vi "AsyncEngine.CANProtectionAndCounter.vi"(10 "Parameters":variant, 11 "Process":refnum<class "Process.lvclass">) -> ()   [LabVIEW 2019, in "Protection and Counter Addon Engine.lvlib"]
uses:
  Protection and Counter Addon Engine.lvlib
  <vilib>/NI/NIVS Inline Async API/_VS Inline Async API/Process/Process.lvclass
  Types/RT Async Engine Settings.ctl
  SubModules/Frame Protection Support/Source/Engine/Types/RT Frame Settings.ctl
  SubModules/Frame Protection Support/Source/Shared/Types/Exported Frame Type.ctl
  SubModules/Frame Protection Support/Source/Engine/Types/RT Protection Configuration.ctl
  SubModules/Frame Protection Support/Source/Shared/Types/Protection Type.ctl
  SubModules/Frame Protection Support/Source/Shared/Types/XNET Signal Configuration.ctl
  SubModules/Frame Protection Support/Source/Shared/Types/Exported Counter Settings.ctl
  SubModules/Frame Protection Support/Source/Shared/Types/Exported Event Trigger Type.ctl
  <vilib>/Platform/TimedLoop/XDataNode/timing_clust.ctl
  <vilib>/Platform/TimedLoop/XDataNode/nitl_modes.ctl
  <vilib>/Platform/TimedLoop/XDataNode/wakeup.ctl
  <vilib>/NI/NIVS Inline Async API/_Data Access Engine/Access Type Classes/Read/Read.lvclass/Read.ctl
  <vilib>/NI/NIVS Inline Async API/_Data Access Engine/Access Type Classes/Write/Write.lvclass/Write.ctl
  <vilib>/NI/NIVS Inline Async API/_VS Inline Async API/Process/Process.lvclass/Process.ctl
  <vilib>/NI/NIVS Inline Async API/_VS Inline Async API/Error Handling Process/SubVIs/Error.ConvertArray.vi
  <vilib>/NI/NIVS Inline Async API/_Data Access Engine/Data Access Engine/Methods/Data.Processes.Execute.vi
  <vilib>/NI/NIVS Inline Async API/_Data Access Engine/Data Access Engine/Methods/Write.Data.vi
  SubModules/Frame Protection Support/Source/Engine/SubVIs/Calculate Counter And Protections Main.vi
  <vilib>/NI/NIVS Inline Async API/_Data Access Engine/Access Type Classes/Write/Write.ProcessData.vi
  <vilib>/NI/NIVS Inline Async API/_Data Access Engine/Data Access Engine/Methods/Read.Data.Detect.vi
  SubModules/Frame Protection Support/Source/Engine/SubVIs/Determine Transmit.vi
  SubModules/Frame Protection Support/Source/Engine/SubVIs/Update Counter Signals.vi
  SubModules/Frame Protection Support/Source/Engine/SubVIs/Get Frame Data.vi
  SubModules/Frame Protection Support/Source/Engine/SubVIs/Convert EU Data to XNET Frame.vi
  SubModules/Frame Protection Support/Source/Engine/SubVIs/Update Protection Signals.vi
  SubModules/Frame Protection Support/Source/Engine/SubVIs/Determine Disabled.vi
  <vilib>/NI/NIVS Inline Async API/_Data Access Engine/Data Access Engine/Methods/Write.Data.Commit.vi
  <vilib>/NI/NIVS Inline Async API/_Data Access Engine/Access Type Classes/Write/Write.Buffer.vi
  <vilib>/NI/NIVS Inline Async API/_Data Access Engine/Access Type Classes/Write/Write.Commit.vi
  <vilib>/NI/NIVS Inline Async API/_Data Access Engine/Access Type Classes/Read/Read.ProcessData.Detect.vi
  SubModules/Frame Protection Support/Source/Engine/SubVIs/Determine Transmission.vi
  SubModules/Frame Protection Support/Source/Engine/SubVIs/Determine Periodic.vi
  SubModules/Frame Protection Support/Source/Engine/SubVIs/Set Counter Signal.vi
  SubModules/Frame Protection Support/Source/Engine/SubVIs/Calculate Counter Value.vi
  SubModules/Frame Protection Support/Source/Engine/SubVIs/Set Protection Signal.vi
  SubModules/Frame Protection Support/Source/Engine/SubVIs/Calculate Protection Value.vi
  <vilib>/NI/NIVS Inline Async API/_Data Access Engine/Data Access Engine/Methods/Write.Data.Buffer.vi
  SubModules/Frame Protection Support/Source/Engine/SubVIs/Get Protection Signals.vi
  <vilib>/xnet/xnet.llb/XNET Convert.vi
  <vilib>/xnet/xnet.llb/XNET Convert (Signal to Frame Raw).vi
  <vilib>/xnet/xnet.llb/XNET Convert (Signal to Frame CAN).vi
  <vilib>/xnet/xnet.llb/XNET Write.vi
  <vilib>/xnet/xnet.llb/XNET Write (Frame CAN).vi
  <vilib>/NI/NI VeriStand Addon Network Comm/Engine/VeriStand Comm.lvclass
  <vilib>/NI/NIVS Inline Async API/_Data Access Engine/Access Type Classes/Write/Write.lvclass
  <vilib>/NI/NIVS Inline Async API/_Data Access Engine/Access Type Classes/Read/Read.lvclass
  <vilib>/Platform/TimedLoop/XDataNode/XDataNode.xnode
  SubModules/Frame Protection Support/Source/Shared/Protection and Counter Support Shared.lvlib
  SubModules/Frame Protection Support/Source/Engine/Protection and Counter Support Engine.lvlib
  <vilib>/Platform/TimedLoop/XDataNode/XDNodeRunTimeDep.lvlib
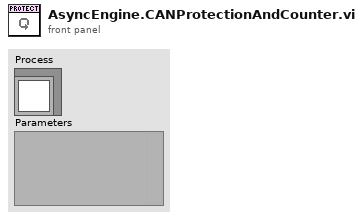
[diagram p1: front panel]
types:
  T1 = typedef "Protection and Counter Addon Engine.lvlib/RT Async Engine Settings.ctl" = cluster{"Name":string, "Priority":i32, "CAN Session":refnum<k21>, "Frame Count":i32, "Frames":T2[], "FPGA Session":u32}
  T2 = typedef "Protection and Counter Support Engine.lvlib/RT Frame Settings.ctl" = cluster{"Type":T3, "Frame ID":u32, "Payload Length":u32, "VS Offset":i32, "VS Length":i32, "Frame Conversion":refnum<k21>, "Frame.Data":dbl[], "Generation Period":u32, "Time Since Last Generation":u32, "Generation Iterations":u32, "Generation Counter":u32, "Has Protection?":bool, "Protection Configurations":T4[], "Has Counter?":bool, "Counter Configurations":T7[], "Has Disable?":bool, "Disable VS Index":i32, "Transmit Trigger":T8, "Trigger VS Index":i32}
  T3 = typedef "Protection and Counter Support Shared.lvlib/Exported Frame Type.ctl" = enum16{"Periodic", "Event", "Periodic/Event"}
  T4 = typedef "Protection and Counter Support Engine.lvlib/RT Protection Configuration.ctl" = cluster{"Protection Frame Index":i32, "Protection Type":T5, "Data Indeces":i32[], "Data Array":dbl[], "Check Sum Conversion":refnum<k21>, "CRC Channels":T6[], "Protection VS Index":i32, "Counter Data Index":i32}
  T5 = typedef "Protection and Counter Support Shared.lvlib/Protection Type.ctl" = enum16{"Arb ID + Bytes Checksum with Inversion", "Arb ID + Bytes CRC with Inversion", "Reversed Raw Signal Checksum with Inversion", "Concatenated Two's Compliment"}
  T6 = typedef "Protection and Counter Support Shared.lvlib/XNET Signal Configuration.ctl" = cluster{"Start Bit":i32, "Name":string, "Number of bits":i32, "Scale":dbl, "Offset":dbl, "Data Type":u32, "Counter":bool}
  T7 = typedef "Protection and Counter Support Shared.lvlib/Exported Counter Settings.ctl" = cluster{"Frame Index":i32, "Max Count":dbl, "VS Index":i32, "Bit Length":i64}
  T8 = typedef "Protection and Counter Support Shared.lvlib/Exported Event Trigger Type.ctl" = enum16{"Channel value change", "Trigger channel (not zero)", "Channel value change or trigger channel (not zero)", "Trigger channel (any value change)", "Channel value change or trigger channel (any value change)"}
  T9 = typedef "Protection and Counter Addon Engine.lvlib/RT Async Engine Variables.ctl" = cluster{"Process Ref":refnum<class "Process.lvclass">, "Comm Ref":refnum<class "VeriStand Comm.lvclass">, "Data Refs":T10, "Settings":T1}
  T10 = typedef "Protection and Counter Addon Engine.lvlib/RT Data References.ctl" = cluster{"ProtectionsAndCounters.Ref":T11, "Signals.Ref":T12, "Status.Ref":T11}
  T11 = typedef "Data Access Engine.lvlib/Data Access Engine.lvclass/Write.DVR.ctl" = refnum<data-value>
  T12 = typedef "Data Access Engine.lvlib/Data Access Engine.lvclass/Read.DVR.ctl" = refnum<data-value>
  T13 = typedef "XDNodeRunTimeDep.lvlib/timing_clust.ctl" = cluster{"Expected End [f-1]":u64, "Actual End [f-1]":u64, "Finished Late? [f-1]":bool, "Expected End [i-1]":u64, "Actual End [i-1]":u64, "Finished Late? [i-1]":bool, "Expected Start [i]":u64, "Actual Start [i]":u64, "Expected Start [f]":u64, "Actual Start [f]":u64, "Source Name":string, "Structure Name":string, "Period":i64, "Deadline":i64, "Offset":i64, "Start":i64, "Priority":i32, "Timeout":i32, "Mode":T14, "Wakeup Reason":T15, "Error":errorcluster, "Source Type":string, "Secondary Source Type":string, "Global End Time":u64, "Global Start Time":u64, "Frame Duration":u64, "Iteration Duration":u64, "Assigned CPU":i32, "I/O Scan Engine Mode":u32}
  T14 = typedef "XDNodeRunTimeDep.lvlib/nitl_modes.ctl" = enum32{"No Change", "Process missed periods, maintain original phase", "Discard missed periods, maintain original phase", "Process missed periods, ignore original phase", "Discard missed periods, ignore original phase"}
  T15 = typedef "XDNodeRunTimeDep.lvlib/wakeup.ctl" = enum32{"Normal", "Aborted", "Asynchronous wakeup", "Timing source error", "Timed loop error", "Timeout"}
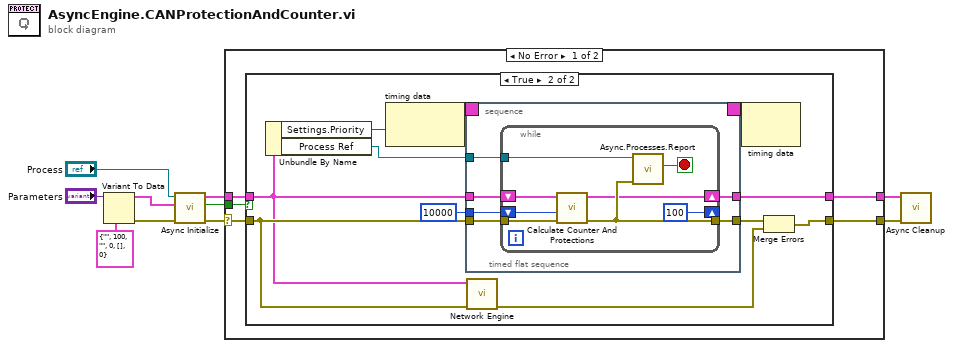
[diagram p0: block diagram]
diagram:
  n1 = Variant To Data(type=T1 {"Name"="", "Priority"=100, "CAN Session"="", "Frame Count"=0, "Frames"=[], "FPGA Session"=0} ("RT Configuration"), Variant="Parameters") -> (data=w2:T1, error out=w5:errorcluster)  [unwired: 1 in]
  n2 = call "Async Initialize.vi"("error in (no error)"=w5, "RT Configuration"=w2, "Process in"="Process") -> ("error out"=w4:errorcluster, "Execute"=w3:bool, "Variables"=w1:T9)  [unwired: 6 in]
  n3 = case shown="No Error" w4 {
    selector: w4 -> [w14 w56]
    tunnel: w3 -> [w15 _]
    tunnel: [w13 w56] -> w6
    tunnel: [w12 w55] -> w7
    tunnel: w1 -> [w11 w55]
    frame No Error {
      n4 = case shown="True" w15 {
        tunnel: w14 -> [w17 w23]
        tunnel: [w17 w19] -> w13
        tunnel: [w16 w28] -> w12
        tunnel: w11 -> [w16 w22]
        frame False {
        }
        frame True {
          n5 = Unbundle By Name(w22) -> ("Settings.Priority"=w25:i32, "Process Ref"=w21:refnum<class "Process.lvclass">)
          n6 = node-c288(w25) -> (w27:T13)
          n7 = timed-sequence {
            timing: w27 -> [_]
            timing-out: [_] -> w26
            tunnel: w21 -> [w30]
            tunnel: w22 -> [w32]
            tunnel: w23 -> [w31]
            tunnel: [w34] -> w24
            tunnel: [w33] -> w28
            tunnel: 10000 ("timeout ms") -> [w29]
            n8 = timed-flat-sequence {
              tunnel: [w36] -> w34
              tunnel: [w37] -> w33
              tunnel: w32 -> [w40]
              tunnel: w31 -> [w39]
              tunnel: w30 -> [w38]
              tunnel: w29 -> [w35]
              n9 = while {
                tunnel: w38 -> [w48]
                tunnel: w39 -> [w47]
                shift-right: [w41] -> w37
                shift-left: w40 -> [w42]
                tunnel: [w45] -> w36
                shift-right: [100 ("timeout ms")] -> _
                shift-left: w35 -> [w44]
                stop <- w46 stop-if-true
                n10 = call "Calculate Counter And Protections.vi"("error in (no error)"=w47, "timeout ms"=w44, "Variables"=w42) -> ("error out"=w45:errorcluster, "Variables out"=w41:T9)  [unwired: 7 in]
                n11 = call <vilib>:"Async.Processes.Report.vi"("Error"=w45, "Process in"=w48) -> ("Stop"=w46:bool)  [unwired: 8 in, 1 out]
              }
            }
          }
          n12 = call "Network Engine.vi"("error in (no error)"=w23, "Variables"=w22) -> ("error out"=w18:errorcluster)  [unwired: 9 in]
          n13 = node-c288(w26) -> ()  [unwired: 1 out]
          n14 = Merge Errors(w24, w18) -> (w19:errorcluster)
        }
      }
    }
    frame Error {
    }
  }
  n15 = call "Async Cleanup.vi"("error in (no error)"=w6, "Variables"=w7) -> ()  [unwired: 9 in, 1 out]
